vi "2-3.vi"() -> ()   [LabVIEW 2022 SP3]
panel:
  in  "确定按钮":bool
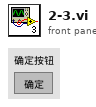
[diagram p1: front panel]
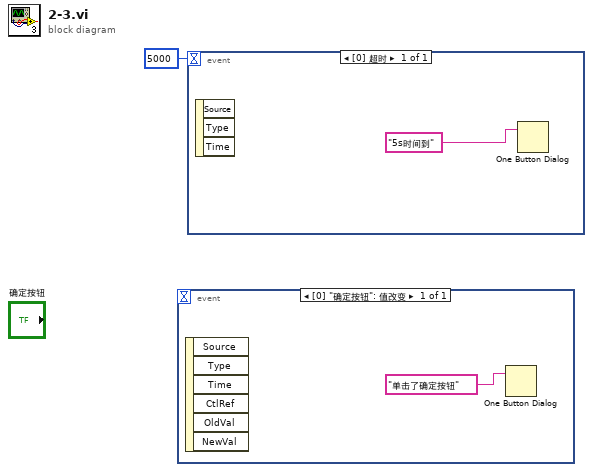
[diagram p0: block diagram]
diagram:
  n1 = event shown="[0] \"确定按钮\": 值改变" {
    selector: _ -> [_]
    dyn-events: _ -> [_]
    timeout: _ -> [_]
    event "确定按钮": Value Change {
      n2 = event-data() -> ()  [unwired: 1 in, 6 out]
      n3 = One Button Dialog(message="单击了确定按钮" ("按钮名称（“确定”）")) -> ()  [unwired: 1 in, 1 out]
    }
  }
  n4 = event shown="[0] 超时" {
    selector: _ -> [_]
    dyn-events: _ -> [_]
    timeout: 5000 -> [_]
    event Timeout {
      n5 = event-data() -> ()  [unwired: 1 in, 3 out]
      n6 = One Button Dialog(message="5s时间到" ("按钮名称（“确定”）")) -> ()  [unwired: 1 in, 1 out]
    }
  }
